vi "Teleop.vi"(10 "Match Info":T1={"Autonomous Elapsed Seconds"=0.0, "TeleOp Elapsed Seconds"=0.0, "Disabled Elapsed Seconds"=0.0, "Visited Autonomous"=FALSE, "Visited TeleOp"=FALSE, "Visited Disabled"=FALSE, "Autonomous Settings"={"Autonomous Style"=enum."Independent", "VI Refnum"=refnum}}, 11 "Call Context":T2) -> ()   [LabVIEW 2019]
doc: "This VI is called for each TeleOp packet received from the DS where the robot is not disabled. It is often used to read from the joysticks and update I/O or to update setpoints for timed control loops. It should complete and return within 20 milliseconds or it may miss DS packets."
uses:
  <vilib>/Rock Robotics/Network Tables/NT Read Boolean.vi
  Robot Global Data.vi
  <vilib>/Rock Robotics/WPI/Joystick/WPI_JoystickArcadeMapping.vi
  <vilib>/Rock Robotics/WPI/ThirdParty/JAS_Junk/TrajLib/Trajectory_Library.lvlib
  <vilib>/Rock Robotics/Network Tables/NT Write Boolean Array.vi
  <vilib>/Rock Robotics/Network Tables/NT Read Number.vi
  <vilib>/Rock Robotics/Network Tables/NT Write Numeric Array.vi
  <vilib>/Rock Robotics/WPI/DriverStation/WPI_DriverStationMatch Info.ctl
  <vilib>/Rock Robotics/WPI/DriverStation/WPI_DriverStationDerivedRobotMode.ctl
panel:
  out "Sample Slider 0":dbl(slide) scale=0.0..5.0
  out "Sample Boolean 1":bool
  out "Sample Boolean 0":bool
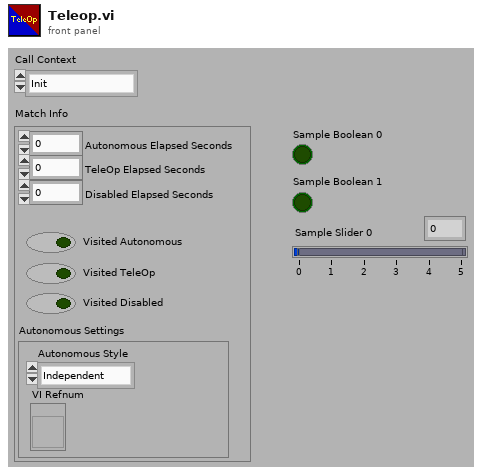
[diagram p1: front panel]
types:
  T1 = typedef "WPI_DriverStationMatch Info.ctl" = cluster{"Autonomous Elapsed Seconds":dbl, "TeleOp Elapsed Seconds":dbl, "Disabled Elapsed Seconds":dbl, "Visited Autonomous":bool, "Visited TeleOp":bool, "Visited Disabled":bool, "Autonomous Settings":cluster{"Autonomous Style":enum16{"Iterative", "Independent"}, "VI Refnum":refnum<vi>}}
  T2 = typedef "WPI_DriverStationDerivedRobotMode.ctl" = enum16{"Init", "Execute", "Stop"}
  T3 = typedef "WPI_JoystickDevRef.ctl" = cluster{"Device":T4}
  T4 = typedef "WPI_JoystickDeviceEnum.ctl" = enum16{"USB 0", "USB 1", "USB 2", "USB 3", "USB 4", "USB 5"}
  T5 = typedef "TRAJ_EXEC_INPUT_SENSORS.ctl" = cluster{"Left Distance":dbl, "Right Distance":dbl, "Gyro Continous\n (inc counterclockwise)":dbl, "Left Speed":dbl, "Right Speed":dbl}
  T6 = typedef "Trajectory_Library.lvlib/RAMSETE.ctl" = cluster{"B":dbl, "Zeta":dbl, "poseTolerance":T7, "poseError":T7, "Enabled":bool}
  T7 = typedef "Trajectory_Library.lvlib/POSE2D.ctl" = cluster{"TRANSLATION":T8, "ROTATION":T9}
  T8 = typedef "Trajectory_Library.lvlib/TRANSLATION2D.ctl" = cluster{"X":dbl, "Y":dbl}
  T9 = typedef "Trajectory_Library.lvlib/ROTATION2D.ctl" = cluster{"VALUE":dbl, "COS":dbl, "SIN":dbl}
  T10 = typedef "Trajectory_Library.lvlib/TRAJ_STATE.ctl" = cluster{"TimeSeconds":dbl, "Velocity":dbl, "Acceleration":dbl, "POSE":T7, "Curvature":dbl}
  T11 = typedef "Trajectory_Library.lvlib/TRANSFORM2D.ctl" = cluster{"TRANSLATION":T8, "ROTATION":T9}
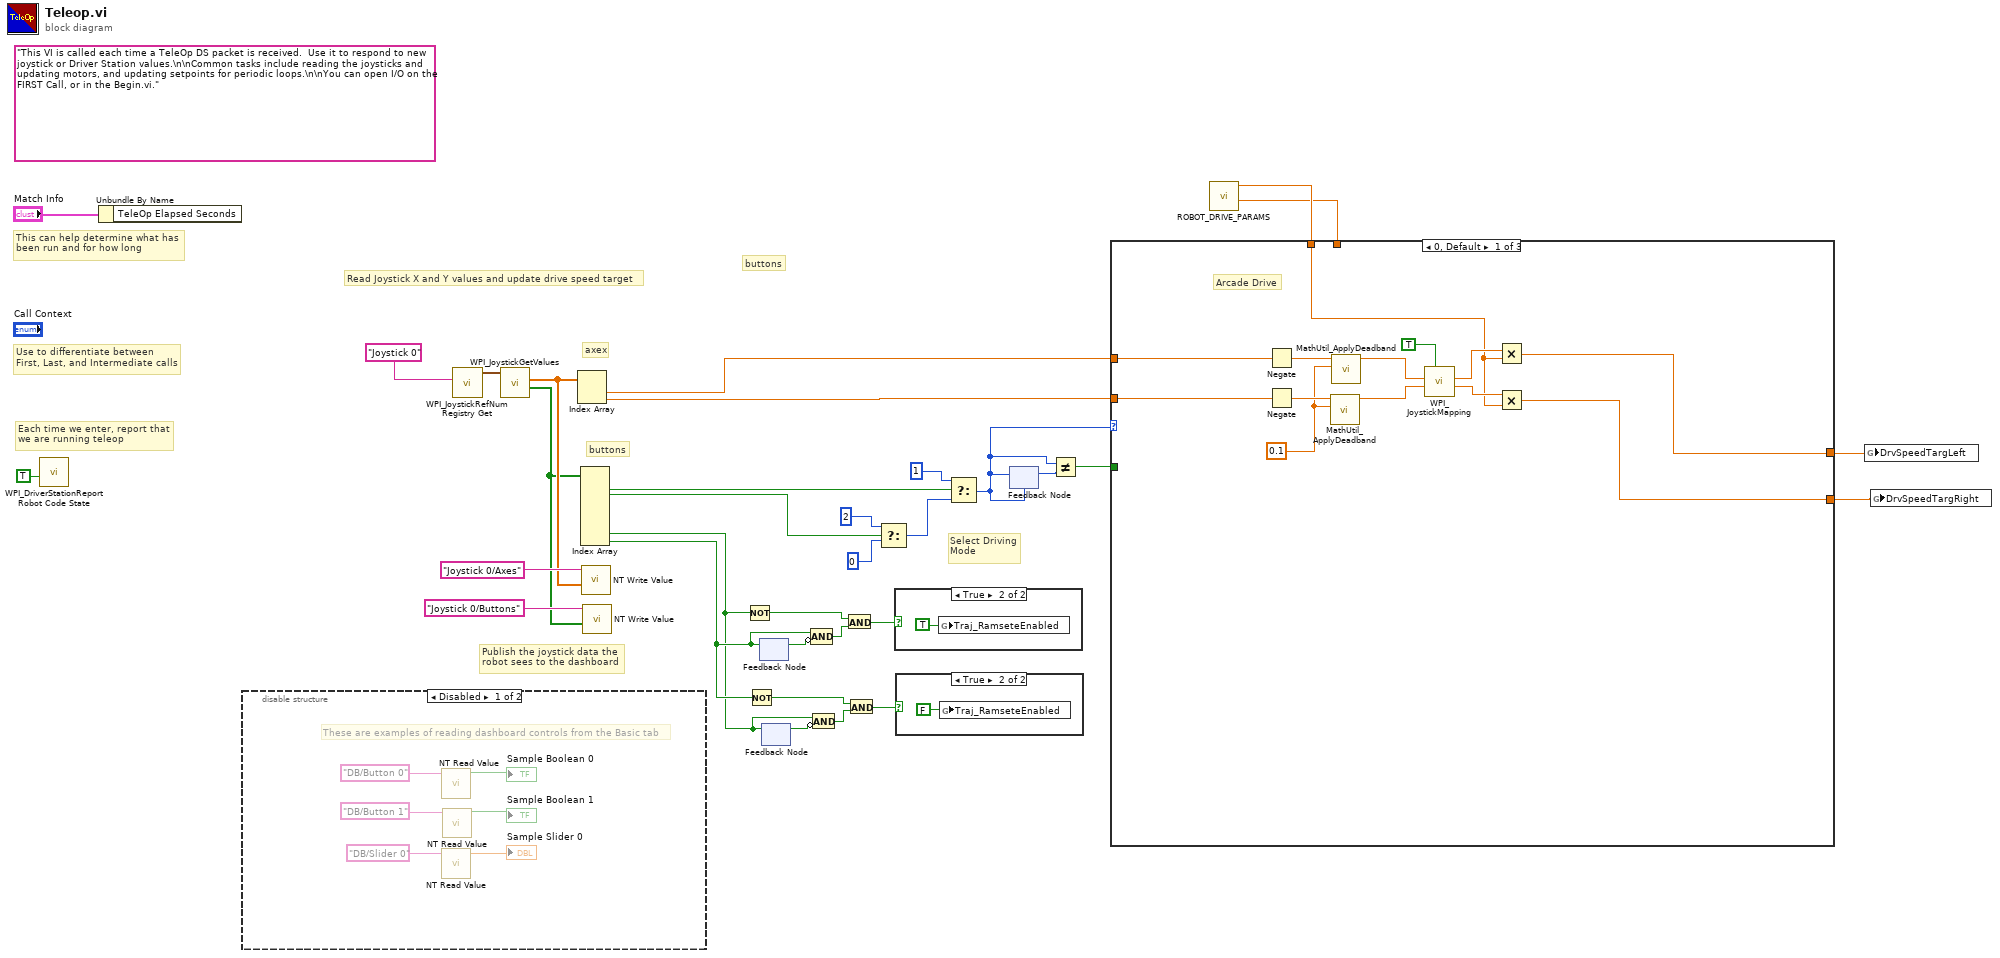
[diagram p0: block diagram]
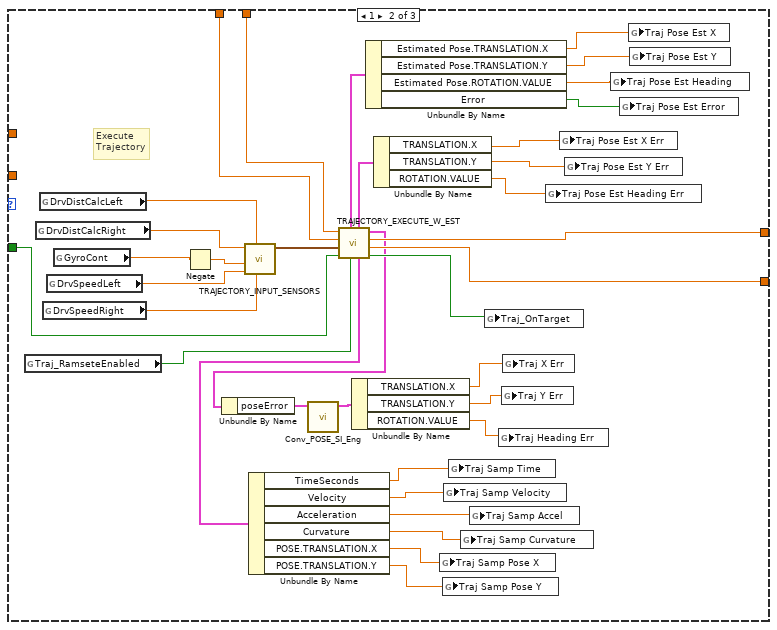
[diagram p4: hidden frame]
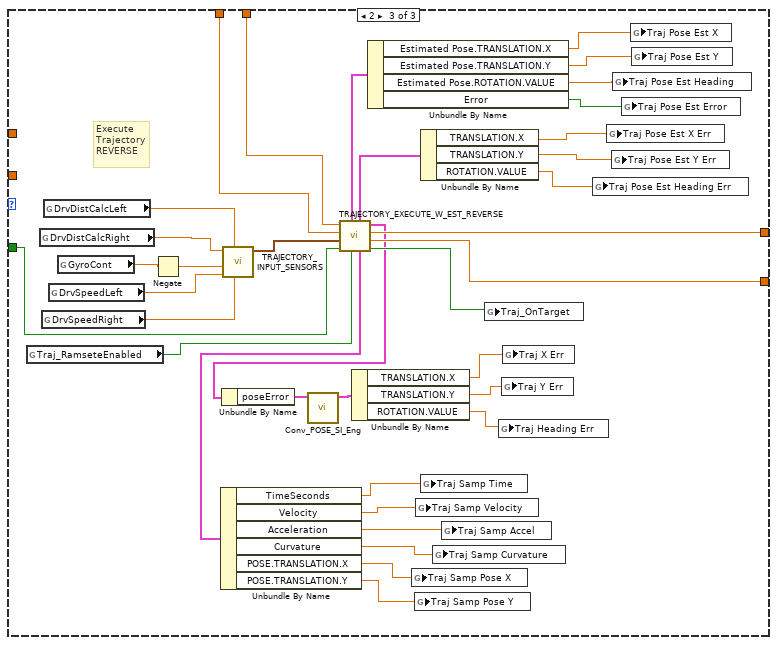
[diagram p5: hidden frame]
diagram:
  (unwired) "This VI is called each time a TeleOp DS packet is received.  Use it to respond to new joystick or Driver Station values.\n\nCommon tasks include reading the joysticks and updating motors, and updating setpoints for periodic loops.\n\nYou can open I/O on the FIRST Call, or in the Begin.vi."
  # "buttons"
  # "Select Driving\nMode"
  # "buttons"
  # "axex"
  # "Publish the joystick data the\nrobot sees to the dashboard"
  # "Each time we enter, report that\nwe are running teleop"
  # "Use to differentiate between\nFirst, Last, and Intermediate calls"
  # "This can help determine what has\nbeen run and for how long"
  # "Read Joystick X and Y values and update drive speed target"
  n1 = call <vilib>:"WPI_DriverStationReport Robot Code State.vi"("TeleOp"=TRUE ("Autonomous")) -> ()  [unwired: 10 in, 1 out]
  n2 = Unbundle By Name("Match Info") -> ()  [unwired: 1 out]
  n3 = disable-structure shown="Disabled" {
    frame Disabled {
      # "These are examples of reading dashboard controls from the Basic tab"
      n4 = call-poly <vilib>:"NT Read Value.vi"("Name"="DB/Button 0" ("refnum name")) -> ("Boolean"=→"Sample Boolean 0":bool)  [unwired: 9 in, 1 out]
      n5 = call-poly <vilib>:"NT Read Value.vi"("Name"="DB/Slider 0" ("refnum name")) -> ("Numeric"=→"Sample Slider 0":dbl)  [unwired: 9 in, 1 out]
      n6 = call-poly <vilib>:"NT Read Value.vi"("Name"="DB/Button 1" ("refnum name")) -> ("Boolean"=→"Sample Boolean 1":bool)  [unwired: 9 in, 1 out]
    }
    frame Enabled {
    }
  }
  n7 = call <vilib>:"WPI_JoystickRefNum Registry Get.vi"("refnum name"="Joystick 0") -> ("JoystickDevRef"=w31:T3)  [unwired: 1 in, 9 out]
  n8 = call <vilib>:"WPI_JoystickGetValues.vi"("JoystickDevRef"=w31) -> ("Buttons"=w21:bool[], "Axes"=w27:dbl[])  [unwired: 6 in, 3 out]
  n9 = Index Array(array=w27) -> (element #1=w26:dbl, element #2=w25:dbl)  [unwired: 2 in]
  n10 = Index Array(array=w21) -> (element #1=w19:bool, element #2=w12:bool, element #7=w1:bool, element #8=w2:bool)  [unwired: 8 in, 4 out]
  n11 = call-poly <vilib>:"NT Write Value.vi"("Numeric Array"=w27, "Name"="Joystick 0/Axes") -> ()  [unwired: 9 in, 1 out]
  n12 = call-poly <vilib>:"NT Write Value.vi"("Boolean Array"=w21, "Name"="Joystick 0/Buttons") -> ()  [unwired: 9 in, 1 out]
  n13 = Not(x=w1) -> (.not. x?=w8:bool)
  n14 = Not(x=w2) -> (.not. x?=w5:bool)
  n15 = feedback #1() -> (w10:bool)  [unwired: 1 in]
  n16 = feedback-in #1(w2) -> ()
  n17 = feedback #2() -> (w7:bool)  [unwired: 1 in]
  n18 = feedback-in #2(w1) -> ()
  n19 = Compound Arithmetic op=AND(w2, invert w10) -> (w9:bool)
  n20 = Compound Arithmetic op=AND(w1, invert w7) -> (w6:bool)
  n21 = And(x=w8, y=w9) -> (x .and. y?=w3:bool)
  n22 = And(x=w5, y=w6) -> (x .and. y?=w4:bool)
  n23 = Select(t=2, s=w12, f=0) -> (s? t:f=w13:i32)
  n24 = case shown="True" w3 {
    frame False {
    }
    frame True {
      n25 = global write "Robot Global Data.vi" "Traj_RamseteEnabled"(TRUE ("Traj_RamseteEnabled")) -> ()
    }
  }
  n26 = case shown="True" w4 {
    frame False {
    }
    frame True {
      n27 = global write "Robot Global Data.vi" "Traj_RamseteEnabled"(FALSE ("Traj_RamseteEnabled")) -> ()
    }
  }
  n28 = Select(t=1, s=w19, f=w13) -> (s? t:f=w17:i32)
  n29 = feedback-in #3(w17) -> ()
  n30 = feedback #3(w17) -> (w18:i32)
  n31 = Not Equal?(x=w17, y=w18) -> (x != y?=w16:bool)
  n32 = call "ROBOT_DRIVE_PARAMS.vi"() -> ("Effective Wheelbase Ft"=w11:dbl, "Max Speed Ft/Sec"=w22:dbl)  [unwired: 10 in]
  n33 = case shown="0, Default" w17 {
    tunnel: w26 -> [w53 _ _]
    tunnel: w25 -> [w52 _ _]
    tunnel: [w51 w89 w125] -> w24
    tunnel: [w50 w88 w124] -> w23
    tunnel: w22 -> [w47 w71 w104]
    tunnel: w16 -> [_ w60 w96]
    tunnel: w11 -> [_ w72 w105]
    frame 0, Default {
      w42 = 0.1 ("Deadband")
      # "Arcade Drive"
      n34 = Negate(x=w53) -> (-x=w45:dbl)
      n35 = Negate(x=w52) -> (-x=w44:dbl)
      n36 = call <vilib>:"MathUtil_ApplyDeadband.vi"("Deadband"=w42, "Value"=w44) -> ("Result"=w43:dbl)  [unwired: 9 in]
      n37 = call <vilib>:"MathUtil_ApplyDeadband.vi"("Deadband"=w42, "Value"=w45) -> ("Result"=w46:dbl)  [unwired: 9 in]
      n38 = call-poly <vilib>:"WPI_JoystickMapping.vi"("Square Inputs"=TRUE, "Y axis value"=w43, "X axis value"=w46) -> ("Right Motor Value"=w48:dbl, "Left Motor Value"=w49:dbl)  [unwired: 7 in]
      n39 = Multiply(x=w49, y=w47) -> (x*y=w51:dbl)
      n40 = Multiply(x=w48, y=w47) -> (x*y=w50:dbl)
    }
    frame 1 {
      # "Execute\nTrajectory"
      n41 = global read "Robot Global Data.vi" "Traj_RamseteEnabled"() -> (w73:bool)
      n42 = global read "Robot Global Data.vi" "DrvDistCalcRight"() -> (w67:dbl)
      n43 = global read "Robot Global Data.vi" "DrvDistCalcLeft"() -> (w66:dbl)
      n44 = global read "Robot Global Data.vi" "DrvSpeedRight"() -> (w68:dbl)
      n45 = global read "Robot Global Data.vi" "DrvSpeedLeft"() -> (w69:dbl)
      n46 = global read "Robot Global Data.vi" "GyroCont"() -> (w90:dbl)
      n47 = Negate(x=w90) -> (-x=w70:dbl)
      n48 = call "TRAJECTORY_INPUT_SENSORS.vi"("Right Speed"=w68, "Left Distance"=w66, "Left Speed"=w69, "Gyro Continous\n (inc counterclockwise)"=w70, "Right Distance"=w67) -> ("Input Sensors"=w65:T5)  [unwired: 6 in]
      n49 = call "TRAJECTORY_EXECUTE_W_EST.vi"("RamseteEnable"=w73, "Init"=w60, "Input Sensors"=w65, "Max Speed\nFT/SEC"=w71, "Wheel Base FT"=w72) -> ("AtReference"=w87:bool, "Right Speed Target"=w88:dbl, "Left Speed Target"=w89:dbl, "outRAMSETE (SI)"=w86:T6, "OutputTRAJ_STATE (SI)"=w74:T10, "Odom Pose Est Diff"=w64:T11, "Pose Est Info"=w55:cluster{"Estimated Pose":T7, "Error":bool})
      n50 = Unbundle By Name(w86) -> ("poseError"=w85:T7)
      n51 = Unbundle By Name(w74) -> ("TimeSeconds"=w80:dbl, "Velocity"=w79:dbl, "Acceleration"=w78:dbl, "Curvature"=w77:dbl, "POSE.TRANSLATION.X"=w76:dbl, "POSE.TRANSLATION.Y"=w75:dbl)
      n52 = call <vilib>:"Conv_POSE_SI_Eng.vi"("Err Pose in SI"=w85) -> ("Err Pose out ENG"=w84:T7)  [unwired: 10 in]
      n53 = Unbundle By Name(w84) -> ("TRANSLATION.X"=w83:dbl, "TRANSLATION.Y"=w82:dbl, "ROTATION.VALUE"=w81:dbl)
      n54 = Unbundle By Name(w55) -> ("Estimated Pose.TRANSLATION.X"=w59:dbl, "Estimated Pose.TRANSLATION.Y"=w58:dbl, "Estimated Pose.ROTATION.VALUE"=w57:dbl, "Error"=w56:bool)
      n55 = Unbundle By Name(w64) -> ("TRANSLATION.X"=w61:dbl, "TRANSLATION.Y"=w62:dbl, "ROTATION.VALUE"=w63:dbl)
      n56 = global write "Robot Global Data.vi" "Traj Samp Pose X"(w76) -> ()
      n57 = global write "Robot Global Data.vi" "Traj Samp Pose Y"(w75) -> ()
      n58 = global write "Robot Global Data.vi" "Traj Samp Velocity"(w79) -> ()
      n59 = global write "Robot Global Data.vi" "Traj Samp Time"(w80) -> ()
      n60 = global write "Robot Global Data.vi" "Traj Samp Curvature"(w77) -> ()
      n61 = global write "Robot Global Data.vi" "Traj Samp Accel"(w78) -> ()
      n62 = global write "Robot Global Data.vi" "Traj_OnTarget"(w87) -> ()
      n63 = global write "Robot Global Data.vi" "Traj Heading Err"(w81) -> ()
      n64 = global write "Robot Global Data.vi" "Traj Y Err"(w82) -> ()
      n65 = global write "Robot Global Data.vi" "Traj X Err"(w83) -> ()
      n66 = global write "Robot Global Data.vi" "Traj Pose Est Heading Err"(w63) -> ()
      n67 = global write "Robot Global Data.vi" "Traj Pose Est X Err"(w61) -> ()
      n68 = global write "Robot Global Data.vi" "Traj Pose Est Y Err"(w62) -> ()
      n69 = global write "Robot Global Data.vi" "Traj Pose Est Heading"(w57) -> ()
      n70 = global write "Robot Global Data.vi" "Traj Pose Est Error"(w56) -> ()
      n71 = global write "Robot Global Data.vi" "Traj Pose Est X"(w59) -> ()
      n72 = global write "Robot Global Data.vi" "Traj Pose Est Y"(w58) -> ()
    }
    frame 2 {
      # "Execute\nTrajectory\nREVERSE"
      n73 = global read "Robot Global Data.vi" "Traj_RamseteEnabled"() -> (w109:bool)
      n74 = global read "Robot Global Data.vi" "DrvDistCalcRight"() -> (w106:dbl)
      n75 = global read "Robot Global Data.vi" "DrvSpeedRight"() -> (w102:dbl)
      n76 = global read "Robot Global Data.vi" "DrvDistCalcLeft"() -> (w107:dbl)
      n77 = global read "Robot Global Data.vi" "DrvSpeedLeft"() -> (w103:dbl)
      n78 = global read "Robot Global Data.vi" "GyroCont"() -> (w126:dbl)
      n79 = Negate(x=w126) -> (-x=w108:dbl)
      n80 = call "TRAJECTORY_INPUT_SENSORS.vi"("Right Speed"=w102, "Left Distance"=w107, "Left Speed"=w103, "Gyro Continous\n (inc counterclockwise)"=w108, "Right Distance"=w106) -> ("Input Sensors"=w101:T5)  [unwired: 6 in]
      n81 = call "TRAJECTORY_EXECUTE_W_EST_REVERSE.vi"("RamseteEnable"=w109, "Init"=w96, "Input Sensors"=w101, "Max Speed\nFT/SEC"=w104, "Wheel Base FT"=w105) -> ("AtReference"=w123:bool, "Right Speed Target"=w124:dbl, "Left Speed Target"=w125:dbl, "outRAMSETE (SI)"=w122:T6, "OutputTRAJ_STATE (SI)"=w110:T10, "Odom Pose Est Diff"=w97:T11, "Pose Est Info"=w95:cluster{"Estimated Pose":T7, "Error":bool})
      n82 = Unbundle By Name(w110) -> ("TimeSeconds"=w116:dbl, "Velocity"=w115:dbl, "Acceleration"=w114:dbl, "Curvature"=w113:dbl, "POSE.TRANSLATION.X"=w112:dbl, "POSE.TRANSLATION.Y"=w111:dbl)
      n83 = Unbundle By Name(w122) -> ("poseError"=w121:T7)
      n84 = call <vilib>:"Conv_POSE_SI_Eng.vi"("Err Pose in SI"=w121) -> ("Err Pose out ENG"=w120:T7)  [unwired: 10 in]
      n85 = Unbundle By Name(w120) -> ("TRANSLATION.X"=w119:dbl, "TRANSLATION.Y"=w118:dbl, "ROTATION.VALUE"=w117:dbl)
      n86 = Unbundle By Name(w95) -> ("Estimated Pose.TRANSLATION.X"=w94:dbl, "Estimated Pose.TRANSLATION.Y"=w93:dbl, "Estimated Pose.ROTATION.VALUE"=w92:dbl, "Error"=w91:bool)
      n87 = global write "Robot Global Data.vi" "Traj Samp Pose X"(w112) -> ()
      n88 = global write "Robot Global Data.vi" "Traj Samp Pose Y"(w111) -> ()
      n89 = global write "Robot Global Data.vi" "Traj Samp Velocity"(w115) -> ()
      n90 = Unbundle By Name(w97) -> ("TRANSLATION.X"=w98:dbl, "TRANSLATION.Y"=w99:dbl, "ROTATION.VALUE"=w100:dbl)
      n91 = global write "Robot Global Data.vi" "Traj Samp Time"(w116) -> ()
      n92 = global write "Robot Global Data.vi" "Traj Samp Curvature"(w113) -> ()
      n93 = global write "Robot Global Data.vi" "Traj Samp Accel"(w114) -> ()
      n94 = global write "Robot Global Data.vi" "Traj_OnTarget"(w123) -> ()
      n95 = global write "Robot Global Data.vi" "Traj Heading Err"(w117) -> ()
      n96 = global write "Robot Global Data.vi" "Traj Y Err"(w118) -> ()
      n97 = global write "Robot Global Data.vi" "Traj X Err"(w119) -> ()
      n98 = global write "Robot Global Data.vi" "Traj Pose Est Heading Err"(w100) -> ()
      n99 = global write "Robot Global Data.vi" "Traj Pose Est X Err"(w98) -> ()
      n100 = global write "Robot Global Data.vi" "Traj Pose Est Y Err"(w99) -> ()
      n101 = global write "Robot Global Data.vi" "Traj Pose Est Heading"(w92) -> ()
      n102 = global write "Robot Global Data.vi" "Traj Pose Est Error"(w91) -> ()
      n103 = global write "Robot Global Data.vi" "Traj Pose Est X"(w94) -> ()
      n104 = global write "Robot Global Data.vi" "Traj Pose Est Y"(w93) -> ()
    }
  }
  n105 = global write "Robot Global Data.vi" "DrvSpeedTargLeft"(w24) -> ()
  n106 = global write "Robot Global Data.vi" "DrvSpeedTargRight"(w23) -> ()
